vi "Day 18-Test.vi"() -> ()   [LabVIEW 2021]
panel:
  in  "String":string
  out "Array out":i32[][](array[numeric])
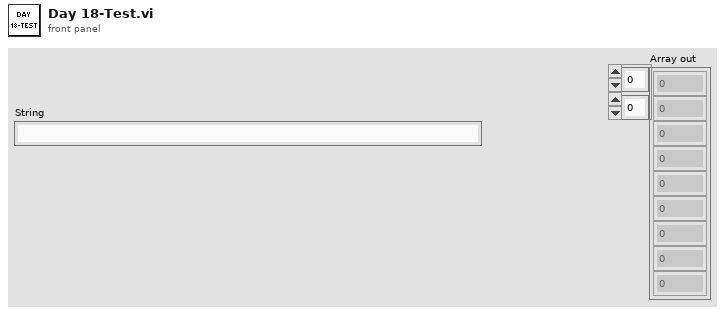
[diagram p1: front panel]
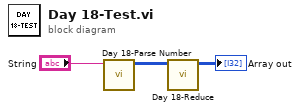
[diagram p0: block diagram]
diagram:
  n1 = call "Day 18-Parse Number.vi"("String"="String") -> ("Array"=w3:i32[][])  [unwired: 10 in]
  n2 = call "Day 18-Reduce.vi"("Array in"=w3) -> ("Array out"=→"Array out":i32[][])  [unwired: 10 in]
